vi "Test_1.vi"(11 "output cluster":T2) -> (3 "RDS Framework.lvlib:RDS Message.lvclass":refnum<class "RDS Message.lvclass">)   [LabVIEW 2015, in "Shore Library.lvlib"]
uses:
  Shore Library.lvlib
  Libraries/RDS Child Messages/MCB/MCB Motor Status.ctl
  Libraries/RDS Framework/RDS Message Class/RDS Message.lvclass
  Libraries/RDS Child Messages/MCB/MCB Channel.ctl
  Libraries/RDS Child Messages/MCB/MCB Status Message/MCB Status.lvclass
  Libraries/RDS Framework/RDS Message ID.ctl
  Libraries/RDS Child Messages/MCB/MCB Status Message/MCB Status.lvclass/MCB Status.ctl
  Libraries/RDS Framework/RDS Message Class/RDS Message.lvclass/RDS Message.ctl
  Libraries/RDS Child Messages/RDS Child Messages.lvlib
panel:
  in  "Motor":T1
  out "Valid?":bool
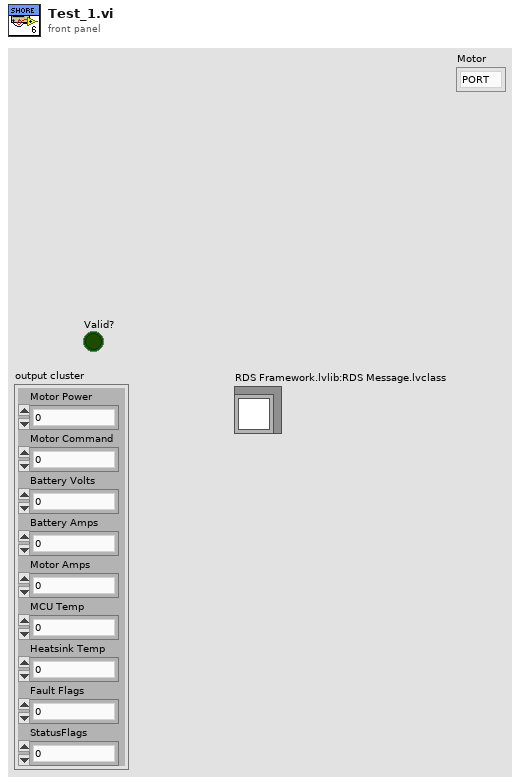
[diagram p1: front panel]
types:
  T1 = typedef "RDS Child Messages.lvlib/MCB Channel.ctl" = enum16{"PORT", "STBD"}
  T2 = typedef "RDS Child Messages.lvlib/MCB Motor Status.ctl" = cluster{"Motor Power":i16, "Motor Command":i16, "Battery Volts":sgl, "Battery Amps":sgl, "Motor Amps":sgl, "MCU Temp":i16, "Heatsink Temp":i16, "Fault Flags":u16, "StatusFlags":u16}
  T3 = typedef "RDS Child Messages.lvlib/RDS Message ID.ctl" = enum16{"RDS Hello World", "String Message", "AIP_Status", "AIP_Command", "GPS_Data", "MCB_Command", "MCB_Status", "Compass_Data", "Depth_Data", "Battery_Data", "Contoller_State", "Set_Mag_Dev", "BTB_Shutdown", "State_Sample_Request", "State_Sample", "PID_Gains_Set", "Helm_Limiter_Set", "Helm_Heading_Command", "Helm_Steering_Command", "Helm_Status", "Controller_Message", "AIP_Set_Min_Depth", "Mission_Controller_State", "Mission_Upload", "Mission_Set_Op_and_Run", "Mission_Settings_Set"}
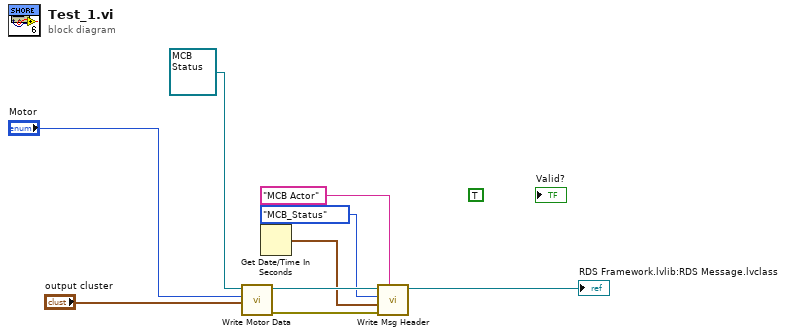
[diagram p0: block diagram]
diagram:
  (unwired) TRUE
  n1 = call "Write Motor Data.vi"("Motor Data"="output cluster", "Motor"="Motor", "MCB Status in"=refnum<class "MCB Status.lvclass"> refnum) -> ("error out"=w4:errorcluster, "MCB Status out"=w8:refnum<class "MCB Status.lvclass">)  [unwired: 7 in]
  n2 = Get Date/Time In Seconds() -> (seconds since 1Jan1904=w5:timestamp)
  n3 = call "Write Msg Header.vi"("Sender Name"="MCB Actor", "error in (no error)"=w4, "Time Stamp"=w5, "Msg ID"=RDS_Message_ID."MCB_Status", "RDS Message in"=w8) -> ("RDS Message out"=→"RDS Framework.lvlib:RDS Message.lvclass":refnum<class "MCB Status.lvclass">)  [unwired: 5 in, 1 out]
